vi "Write_parameter.vi"(8 "error in (no error)":errorcluster caption="entrée d'erreur (pas d'erreur)", 10 "Parameter":string, 11 "Class DIO en entrée":refnum<class "Class Instrument DIO.lvclass">) -> (0 "error out":errorcluster caption="sortie d'erreur", 3 "Class DIO en Sortie":refnum<class "Class Instrument DIO.lvclass">)   [LabVIEW 2020, in "Library Instrument & Equipement.lvlib" / "Library Instruments.lvlib" / "Class Instrument DIO.lvclass"]
uses:
  Class Instrument DIO.lvclass
  Commun VI/TypeDef/Commande DIO/Parameter DIO.ctl
  DIO/Class DIO (Default)/Class DIO (Default).lvclass
  JSON API/JSON Value/Set from JSON string.vi
  Instrument (Default)/Class Instrument (Default).lvclass
  JSON API/JSON Value/JSON Value.lvclass
  Class Instrument DIO.lvclass/Class Instrument DIO.ctl
  JSON API/Variant JSON/Variant JSON.lvlib
  JSON API/Get Polymorphic/JSON GetSet.lvlib
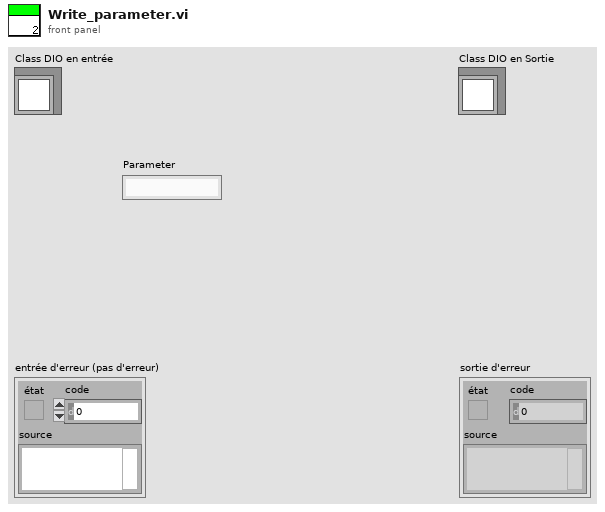
[diagram p1: front panel]
types:
  T1 = typedef "Parameter DIO.ctl" = cluster{"Device_Com_Port":string, "Port":u8, "Line":u8, "Function":enum16{"Write", "Read"}, "Class DIO":refnum<class "Class DIO (Default).lvclass">}
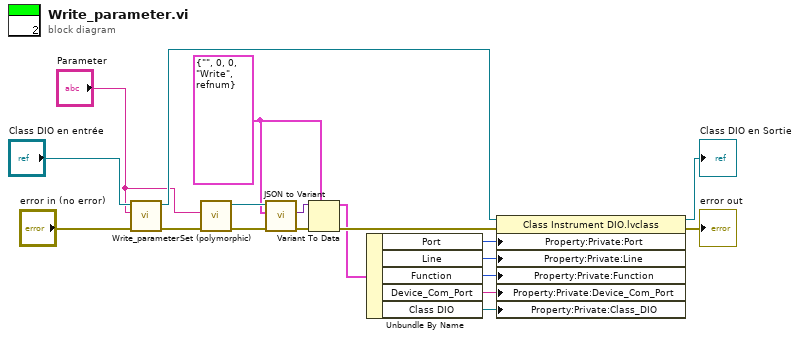
[diagram p0: block diagram]
diagram:
  w8 = T1 {"Device_Com_Port"="", "Port"=0, "Line"=0, "Function"=enum."Write", "Class DIO"=refnum} ("Parameter")
  n1 = call-parent "Write_parameter.vi"("error in (no error)"="error in (no error)", "Parameter"="Parameter", "Class Instrument (Default) en entrée"="Class DIO en entrée") -> ("error out"=w7:errorcluster, "Class Instrument (Default) en sortie"=w5:refnum<class "Class Instrument DIO.lvclass">)  [unwired: 7 in]
  n2 = call-poly "Set (polymorphic).vi"("error in (no error)"=w7, "JSON stream"="Parameter") -> ("error out"=w17:errorcluster, "JSON Value out"=w19:refnum<class "JSON Value.lvclass">)  [unwired: 7 in, 1 out]
  n3 = call "JSON to Variant.vi"("error in (no error)"=w17, "Variant (Data Type)"=w8, "JSON Value"=w19) -> ("error out"=w18:errorcluster, "Variant out"=w16:variant)  [unwired: 7 in]
  n4 = Variant To Data(error in=w18, type=w8, Variant=w16) -> (data=w11:T1, error out=w12:errorcluster)
  n5 = Unbundle By Name(w11) -> ("Port"=w9:u8, "Line"=w10:u8, "Function"=w3:enum16{"Write", "Read"}, "Device_Com_Port"=w2:string, "Class DIO"=w1:refnum<class "Class DIO (Default).lvclass">)
  n6 = property class="Class Instrument DIO.lvclass"(reference=w5, error in=w12, "Property:Private:Port"=w9, "Property:Private:Line"=w10, "Property:Private:Function"=w3, "Property:Private:Device_Com_Port"=w2, "Property:Private:Class_DIO"=w1) -> (reference out=→"Class DIO en Sortie":refnum<class "Class Instrument DIO.lvclass">, error out=→"error out":errorcluster)
